vi "poly_eval_vector.vi"(2 "P(x)":dbl[](array[numeric]) min=0.0 max=127.0 format="%#.2f", 3 "A":dbl[](array[numeric])) -> (1 "P(A)":dbl[](array[numeric]))   [LabVIEW 2020]
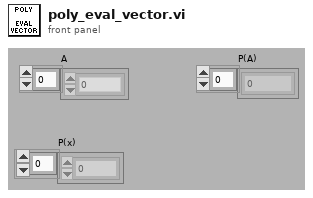
[diagram p1: front panel]
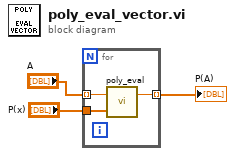
[diagram p0: block diagram]
diagram:
  n1 = for {
    tunnel: "P(x)" -> [w6]
    tunnel: "A" -> [w5] mode=indexing
    tunnel: [w4] -> w1 mode=indexing
    n2 = call "poly_eval.vi"("P(x)"=w6, "A"=w5) -> ("P(A)"=w4:dbl)  [unwired: 1 in]
  }
  "P(A)" <- w1
